vi "ExtWriteBonTriton.vi"() -> ()   [LabVIEW 2016]
panel:
  in  "Tab Control 2":enum32{"Settings", "Operstion"}(tab)
  in  "B_present Channel":i32
  in  "Maximum trial":i32=2
  in  "B_target channel":i32
  out "B target (T)":dbl
  out "B Present (T)":dbl
  in  "Reinitialize":bool
  in  "Rate (per min)":dbl=0.1
  out "status":string
  in  "ON?":bool
  out "error out":errorcluster
  in  "Boolean":bool
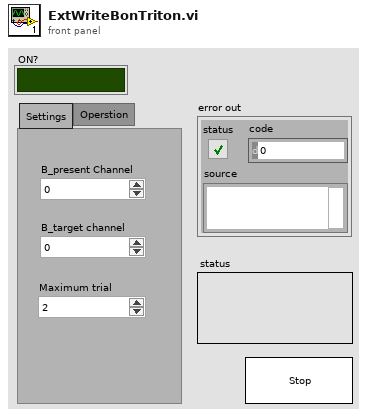
[diagram p1: front panel]
types:
  T1 = enum16{"Read", "Write", "ReadWrite", "BufferedRead", "BufferedReadWrite"}
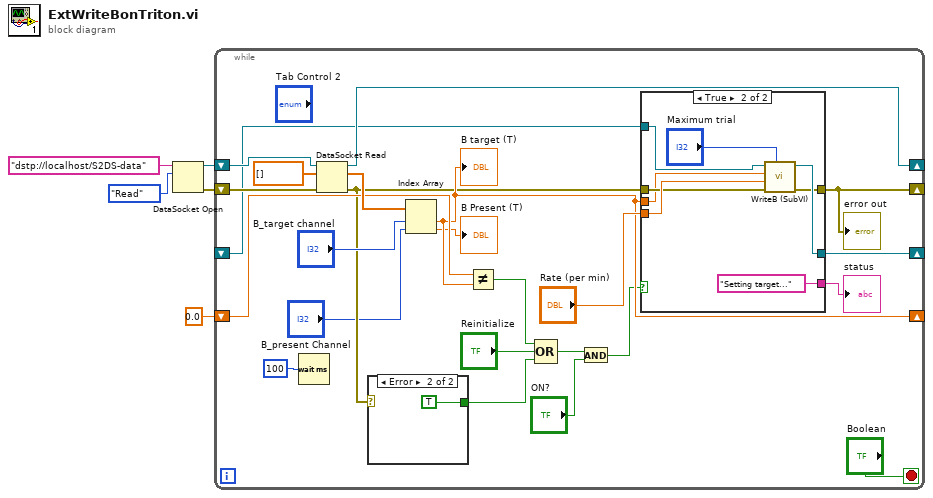
[diagram p0: block diagram]
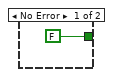
[diagram p2: hidden frame]
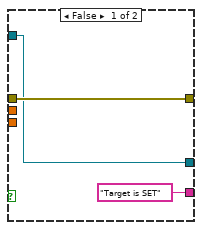
[diagram p3: hidden frame]
diagram:
  n1 = DataSocket Open(10:T1."Read" ("mode"), 11:"dstp://localhost/S2DS-data" ("URL")) -> (0:w2:errorcluster, 3:w3:refnum<k13>)  [unwired: 2 in]
  n2 = while {
    shift-right: [w26] -> _
    shift-left: w3 -> [w28]
    shift-right: [w20] -> _
    shift-left: w2 -> [w29]
    shift-right: [w21] -> _
    shift-left: _ -> [w19]
    shift-right: [w16] -> _
    shift-left: 0.0 -> [w17]
    stop <- "Boolean" stop-if-true
    n3 = Wait (ms)(milliseconds to wait=u32 100) -> ()  [unwired: 1 out]
    n4 = DataSocket Read(8:w29, 10:dbl[] [], 11:w28) -> (0:w13:errorcluster, 2:w23:dbl[], 3:w26:refnum<k13>)  [unwired: 2 in, 4 out]
    n5 = case shown="Error" w13 {
      tunnel: [FALSE TRUE] -> w12
      frame No Error {
      }
      frame Error {
      }
    }
    n6 = Index Array(array=w23, index #1="B_target channel", index #2="B_present Channel") -> (element #1=w16:dbl, element #2=→"B Present (T)":dbl)
    "B target (T)" <- w16
    n7 = Not Equal?(x=w17, y=w16) -> (x != y?=w15:bool)
    n8 = Compound Arithmetic op=OR(w15, "Reinitialize", w12) -> (w11:bool)
    n9 = And(x=w11, y="ON?") -> (x .and. y?=w10:bool)
    n10 = case shown="True" w10 {
      tunnel: [w33 w42] -> w21
      tunnel: [w34 w41] -> w20
      tunnel: w19 -> [w33 w40]
      tunnel: "Rate (per min)" -> [_ w39]
      tunnel: w13 -> [w34 w37]
      tunnel: w16 -> [_ w36]
      tunnel: ["Target is SET" ("String") "Setting target..." ("String")] -> w8
      frame False {
      }
      frame True {
        n11 = call "WriteB (SubVI).vi"("Try"="Maximum trial", "error IO"=w37, "Sweep rate"=w39, "Target B"=w36, "VISA resource name"=w40) -> ("error out"=w41:errorcluster, "VISA Refnum out"=w42:refnum<visa-resource-name>)  [unwired: 5 in]
      }
    }
    "error out" <- w20
    "status" <- w8
  }
